vi "Data_get.vi"() -> ()   [LabVIEW 2009]
uses:
  <vilib>/Analysis/2dsp.llb/Real FFT.vi
  <vilib>/Analysis/NI_AALPro.lvlib
panel:
  in  "#steps":u32=1 min=1
  in  "f step (MHz)":dbl=0.0003 min=0.00025 max=67.0 step=1e-06 format="%#.12f"
  in  "ps/point":T1(ring)
  in  "ns/div":T2(ring)
  out "Current sweep":u32=1 min=1 max=1000 step=1
  in  "Ext":string="ccd"
  out "f cur. (MHz)":string
  in  "Name":string="trace"
  in  "Folder":path
  in  "#Sweeps":u32=1 min=1 max=1000 step=1
  in  "Ampl. (dBm)":dbl min=-135.0 max=30.0 step=0.5 format="%#_8g"
  in  "f start (MHz)":dbl=0.0003 min=0.00025 max=67.0 step=1e-06 format="%#.12f"
  in  "Start":bool
  in  "Quit":bool
  in  "E8257D VISA Port":refnum<visa-resource-name>="GPIB0::1::INSTR"
  out "read time (ms)":u32
  out "#points":u32
  out "Busy":bool
  in  "Repetition rate (Hz)":ext=2.5
  in  "Chirp start (MHz)":ext=2.5
  in  "Filter up to (MHz)":ext=2.5
  in  "Amount of averagings":u32=10
  out "Data":dbl[](array[numeric])
  out "XY Graph 5":cluster{ext[], dbl[]}(graph)
  out "FFT (Im)":dbl[](array[numeric])
  out "FFT (Re)":dbl[](array[numeric])
  out "Final array":ext[][](array[numeric])
  out "size(s)":i32
  out "Oscilloscope Data":dbl[](array[numeric])
  in  "Channel Number":u16=1
  out "Oscilloscope graph":dbl[](graph)
  in  "Stop":bool
  in  "TDS VISA Port":refnum<visa-resource-name>="GPIB0::1::INSTR"
  # "TDS6000"
  # "E8257D"
  # "File Storage"
  # "Control"
  # "Spectrum data"
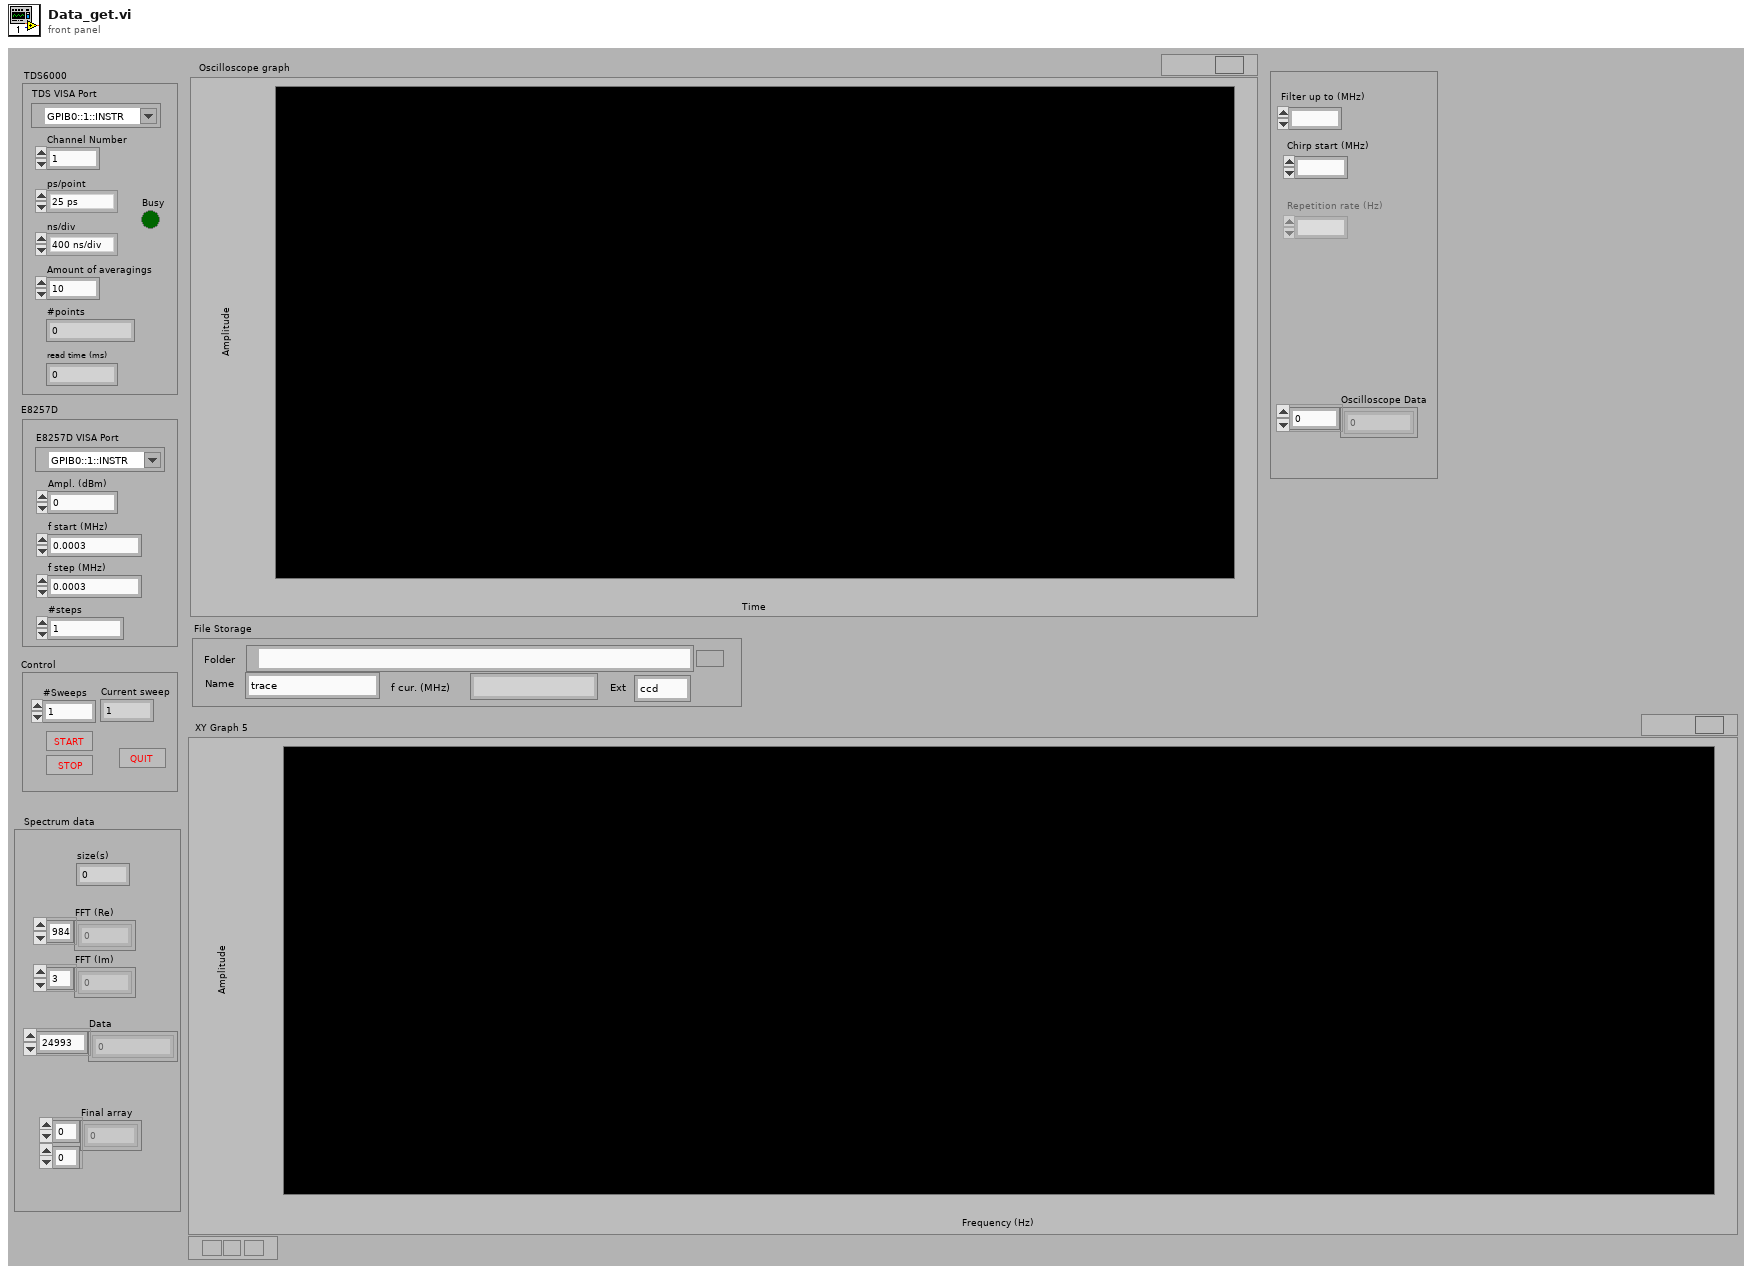
[diagram p1: front panel]
types:
  T1 = enum16{"25 ps", "50 ps", "100 ps", "200 ps", "400 ps", "800 ps", "2 ns"}
  T2 = enum16{"400 ns/div", "1 us/div", "2 us/div", "4 us/div", "10 us/div", "20 us/div"}
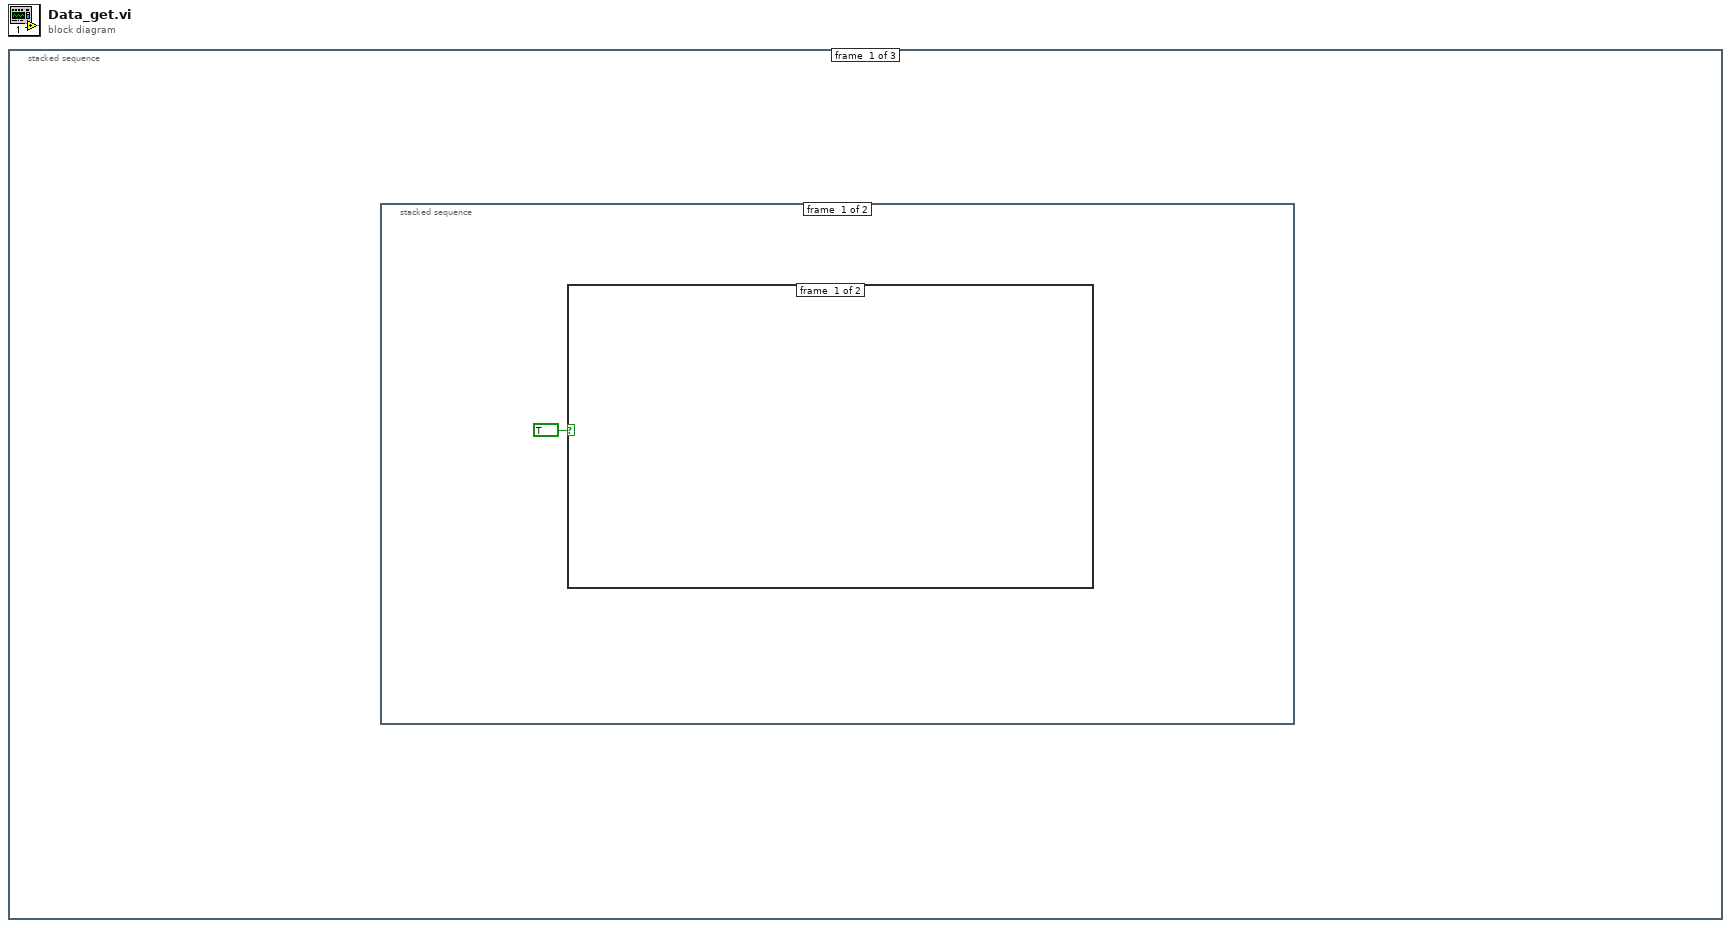
[diagram p0: block diagram]
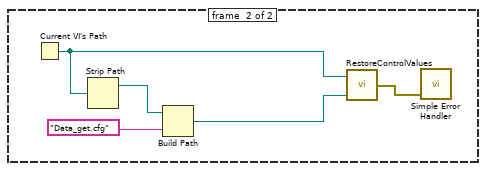
[diagram p2: hidden frame]
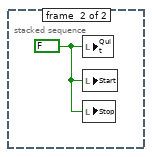
[diagram p3: hidden frame]
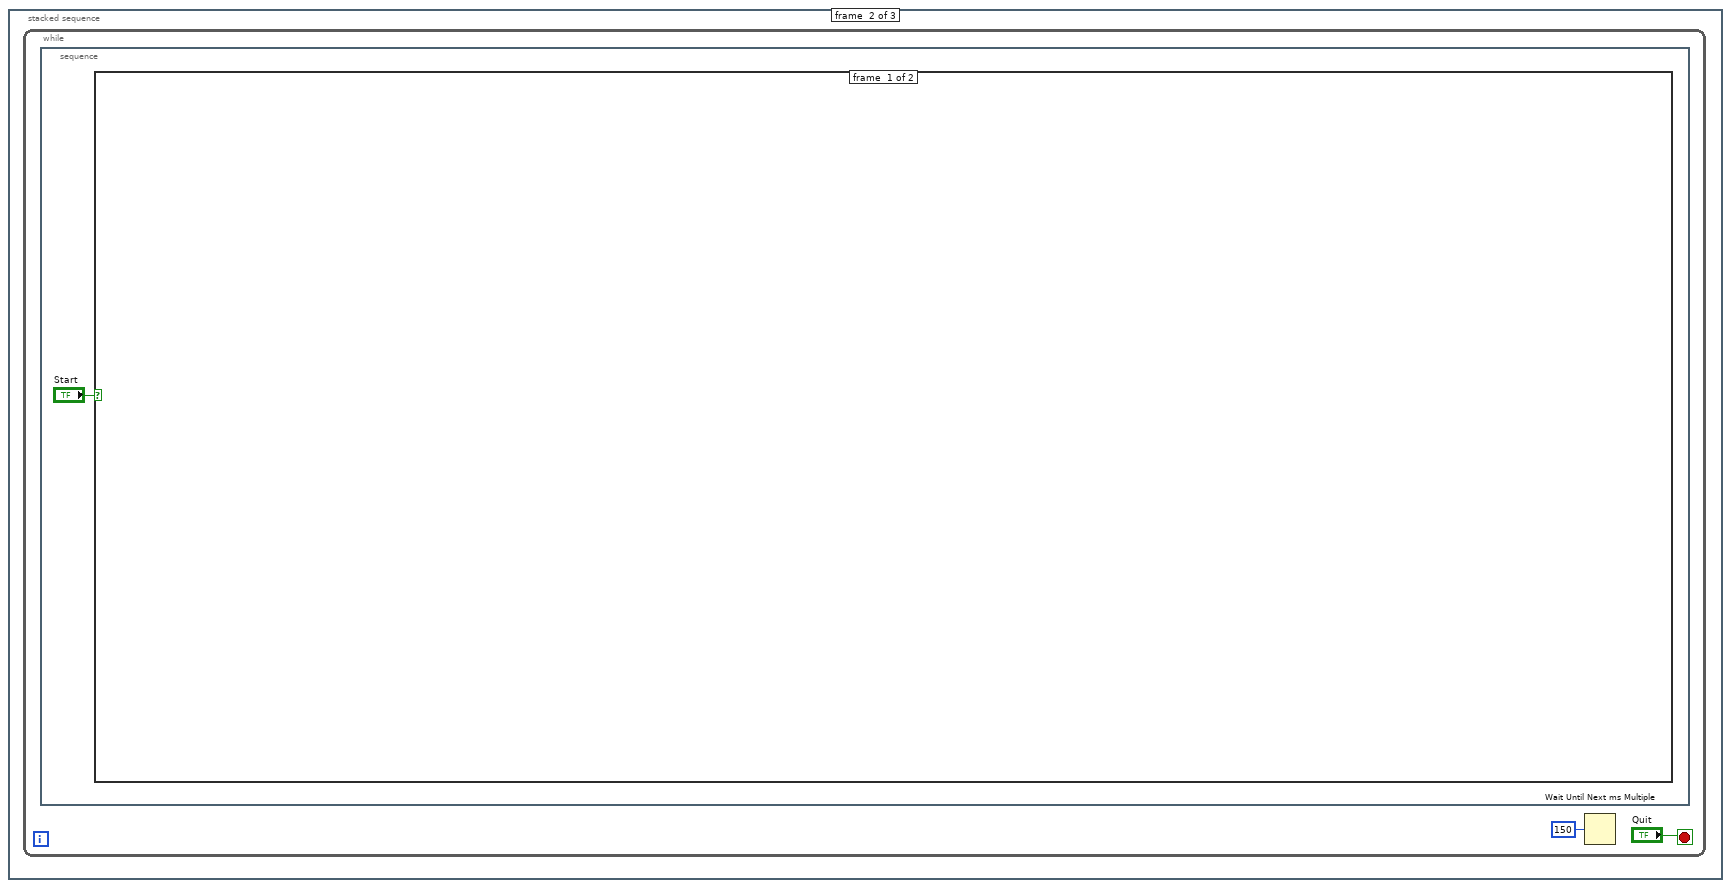
[diagram p4: hidden frame]
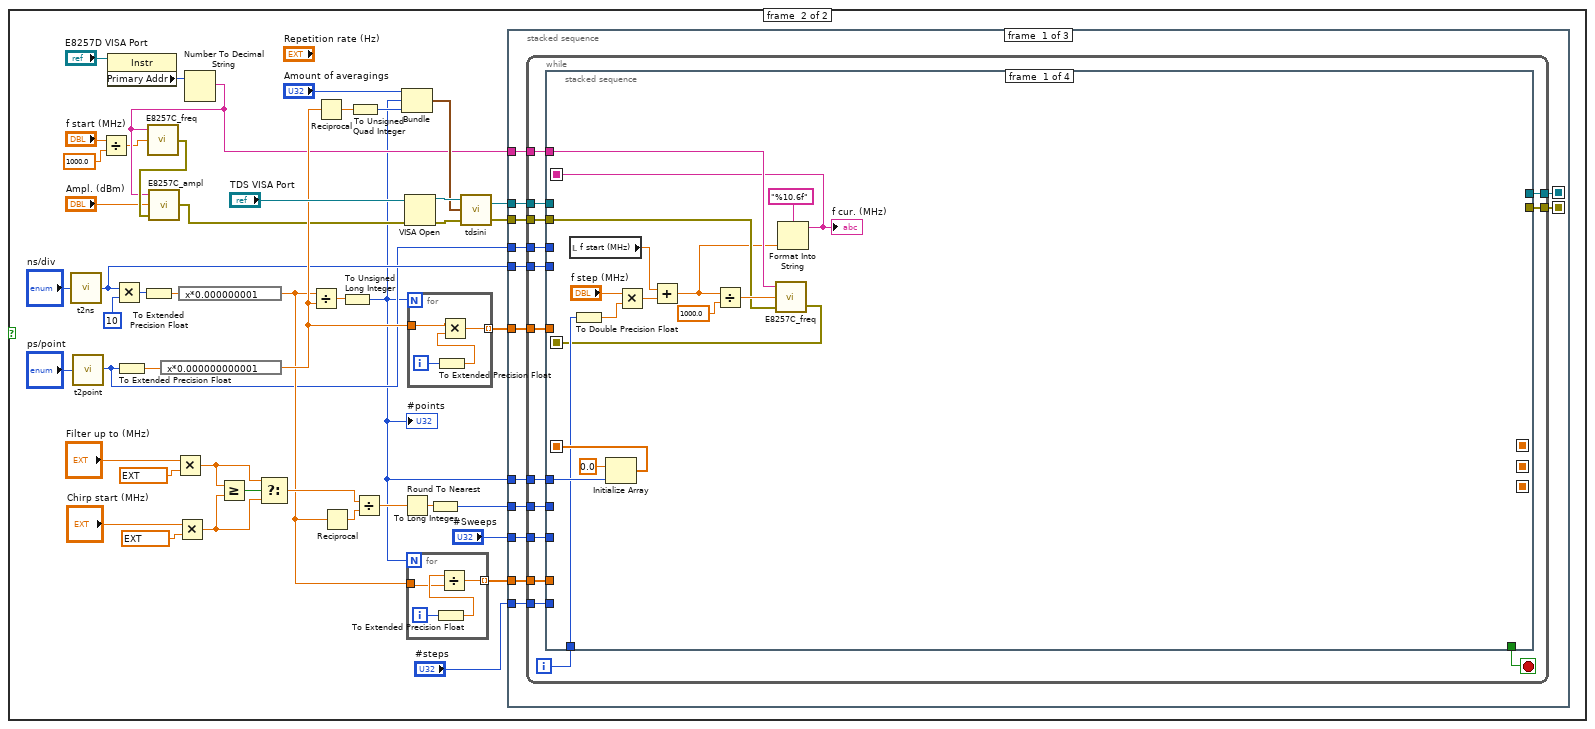
[diagram p5: hidden frame]
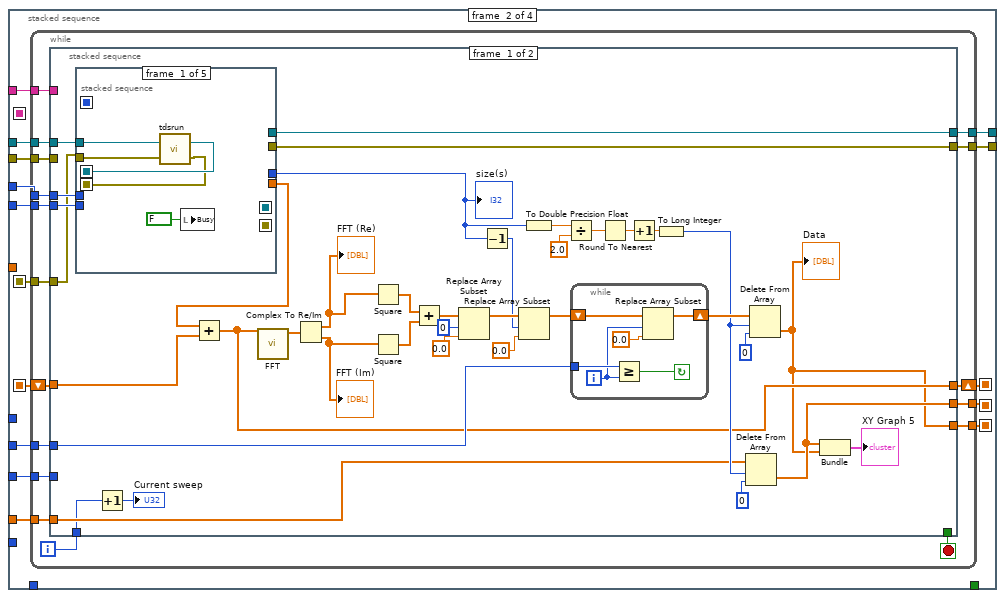
[diagram p6: hidden frame]
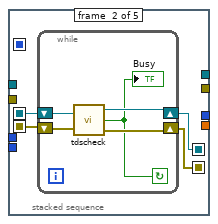
[diagram p7: hidden frame]
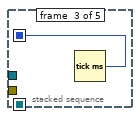
[diagram p8: hidden frame]
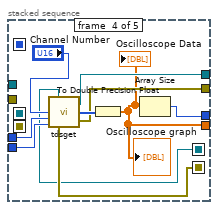
[diagram p9: hidden frame]
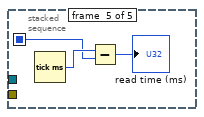
[diagram p10: hidden frame]
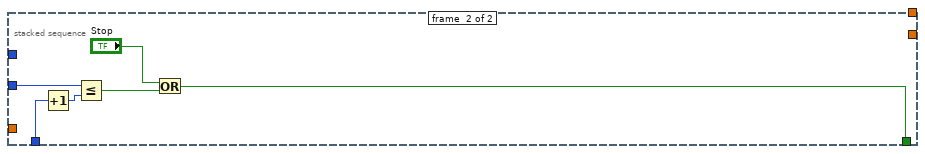
[diagram p11: hidden frame]
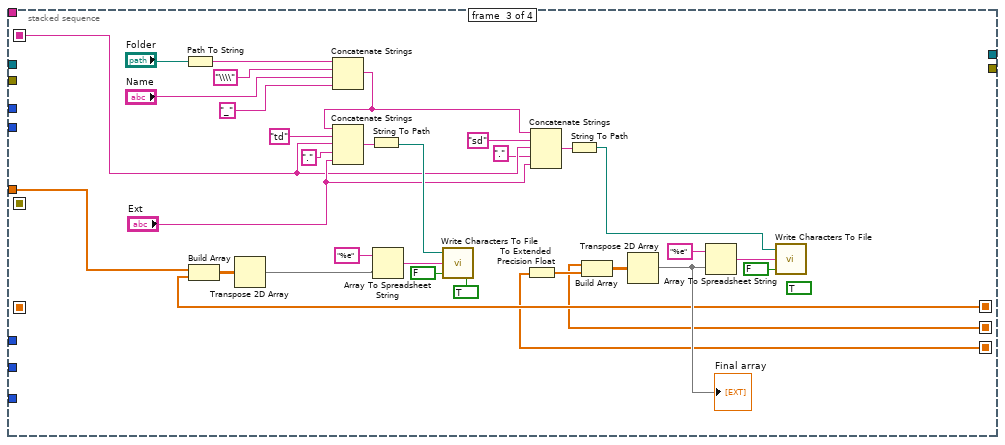
[diagram p12: hidden frame]
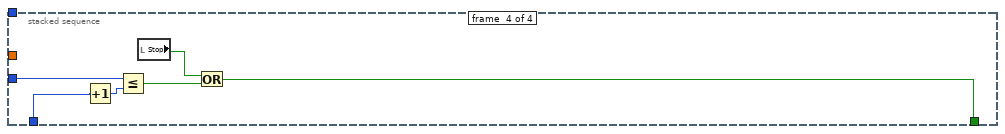
[diagram p13: hidden frame]
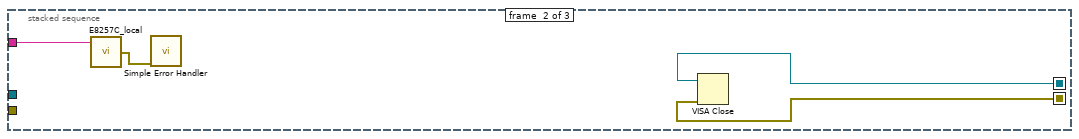
[diagram p14: hidden frame]
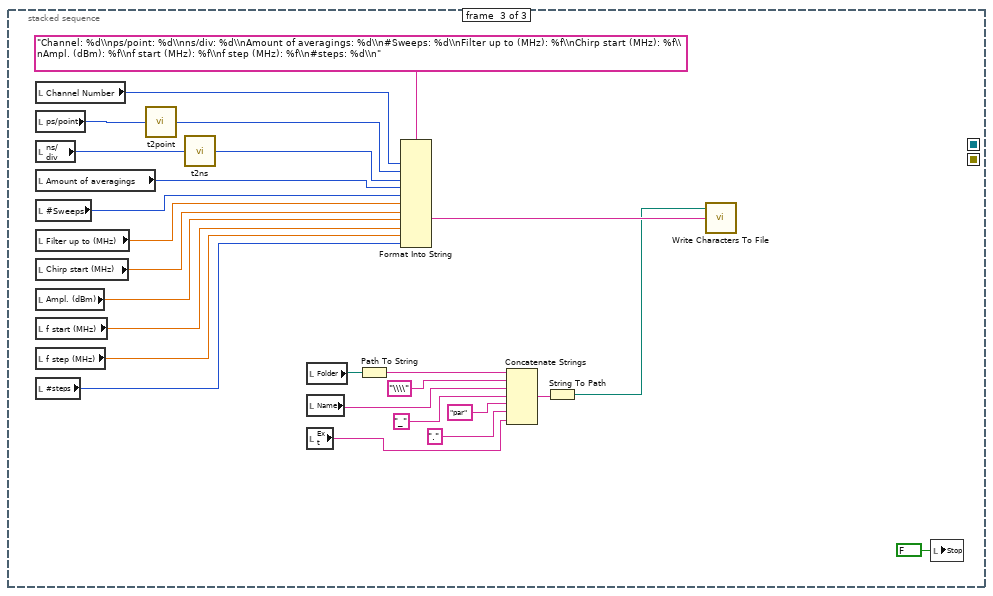
[diagram p15: hidden frame]
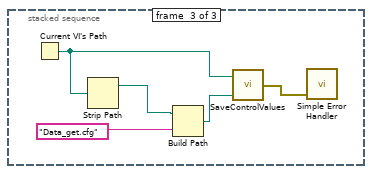
[diagram p16: hidden frame]
diagram:
  n1 = stacked-sequence {
    frame #0 {
      n2 = stacked-sequence {
        frame #0 {
          n3 = case shown="True" TRUE {
            frame #0 {
            }
            frame #1 {
              n4 = Current VI's Path() -> (path=w2:path)
              n5 = Strip Path(path=w2) -> (stripped path=w3:path)  [unwired: 1 out]
              n6 = Build Path(base path=w3, name or relative path="Data_get.cfg") -> (appended path=w5:path)
              n7 = call "RestoreControlValues.vi"("file path"=w5, "vi path"=w2) -> ("error out"=w4:errorcluster)
              n8 = call <vilib>:"Simple Error Handler.vi"("error in (no error)"=w4) -> ()  [unwired: 4 in, 5 out]
            }
          }
        }
        frame #1 {
          w7 = FALSE ("Quit")
          n9 = local write "Quit"(w7) -> ()
          n10 = local write "Start"(w7) -> ()
          n11 = local write "Stop"(w7) -> ()
        }
      }
    }
    frame #1 {
      n12 = while {
        stop <- "Quit" stop-if-true
        n13 = stacked-sequence {
          frame #0 {
            n14 = case shown="True" "Start" {
              frame #0 {
              }
              frame #1 {
                n15 = call "t2ns.vi"("t/div"="ns/div") -> ("ns/div"=w16:u32)
                n16 = call "t2point.vi"("t/point"="ps/point") -> ("ps/point"=w14:u32)
                n17 = Divide(x="f start (MHz)", y=1000.0) -> (x/y=w19:dbl)
                n18 = property class="Instr"(reference="E8257D VISA Port") -> ("Primary Addr"=w26:u16)  [unwired: 1 in, 2 out]
                n19 = Multiply(x=w16, y=u32 10) -> (x*y=w50:u32)
                n20 = To Extended Precision Float(1:w14) -> (0:w47:ext)
                n21 = To Extended Precision Float(1:w50) -> (0:w48:ext)
                n22 = expression code="x*0.000000000001"(w47) -> (w32:ext)
                n23 = Multiply(x="Filter up to (MHz)", y=ext 1000000.0) -> (x*y=w38:ext)
                n24 = Multiply(x="Chirp start (MHz)", y=ext 1000000.0) -> (x*y=w35:ext)
                n25 = expression code="x*0.000000001"(w48) -> (w28:ext)
                n26 = Number To Decimal String(number=w26) -> (decimal integer string=w23:string)  [unwired: 1 in]
                n27 = call "E8257C_freq.vi"("Frequency GHz"=w19, "GPIB address"=w23) -> ("error out"=w24:errorcluster)  [unwired: 1 in]
                n28 = call "E8257C_ampl.vi"("error in"=w24, "Amplitude dBm"="Ampl. (dBm)", "GPIB address"=w23) -> ("error out"=w22:errorcluster)
                n29 = Greater Or Equal?(x=w38, y=w35) -> (x >= y?=w46:bool)
                n30 = Select(t=w38, s=w46, f=w35) -> (s? t:f=w44:ext)
                n31 = Divide(x=w28, y=w32) -> (x/y=w49:ext)
                n32 = Reciprocal(x=w32) -> (1/x=w30:ext)
                n33 = Reciprocal(x=w28) -> (1/x=w45:ext)
                n34 = To Unsigned Long Integer(number=w49) -> (unsigned 32bit integer=w12:u32)
                "#points" <- w12
                n35 = To Unsigned Quad Integer(1:w30) -> (0:w31:u64)
                n36 = Divide(x=w44, y=w45) -> (x/y=w43:ext)
                n37 = Bundle("Amount of averagings"="Amount of averagings", w12, w31) -> (w33:cluster{"Amount of averagings ":u32, u32, u64})  [unwired: 1 in]
                n38 = Round To Nearest(number=w43) -> (nearest integer value=w42:ext)
                n39 = VISA Open(error in (no error)=w22, VISA resource name="TDS VISA Port") -> (VISA resource name=w53:refnum<visa-resource-name>, error out=w54:errorcluster)  [unwired: 3 in]
                n40 = for {
                  N: w12 -> [_]
                  tunnel: w28 -> [w279]
                  tunnel: [w281] -> w29 mode=indexing
                  i -> [w282]
                  n41 = To Extended Precision Float(1:w282) -> (0:w280:ext)
                  n42 = Divide(x=w280, y=w279) -> (x/y=w281:ext)
                }
                n43 = for {
                  N: w12 -> [_]
                  tunnel: w32 -> [w284]
                  tunnel: [w283] -> w17 mode=indexing
                  i -> [w286]
                  n44 = To Extended Precision Float(1:w286) -> (0:w285:ext)
                  n45 = Multiply(x=w284, y=w285) -> (x*y=w283:ext)
                }
                n46 = To Long Integer(number=w42) -> (32bit integer=w41:i32)
                n47 = call "tdsini.vi"("Error In (No Error)"=w54, "Acq_par"=w33, "VISA Port In"=w53) -> ("Error Out"=w55:errorcluster, "VISA Port Out"=w56:refnum<visa-resource-name>)
                n48 = stacked-sequence {
                  seq-local: [w61 _ _] -> [_ w252 _]
                  seq-local: [w60 _ _] -> [_ w251 _]
                  tunnel: w56 -> [w69 _ _]
                  tunnel: w55 -> [w68 _ _]
                  tunnel: w14 -> [w67 _ _]
                  tunnel: w16 -> [w66 _ _]
                  tunnel: w41 -> [w65 _ _]
                  tunnel: w29 -> [w64 _ _]
                  tunnel: w23 -> [w63 w249 _]
                  tunnel: "#Sweeps" -> [w62 _ _]
                  tunnel: w17 -> [w57 _ _]
                  tunnel: w12 -> [w59 _ _]
                  tunnel: "#steps" -> [w58 _ _]
                  frame #0 {
                    n49 = while {
                      tunnel: w69 -> [w84]
                      tunnel: w68 -> [w83]
                      tunnel: w67 -> [w82]
                      tunnel: w66 -> [w81]
                      tunnel: w65 -> [w80]
                      tunnel: w64 -> [w79]
                      tunnel: w63 -> [w78]
                      tunnel: w62 -> [w77]
                      tunnel: [w76] -> w61
                      tunnel: [w75] -> w60
                      tunnel: w59 -> [w74]
                      tunnel: w58 -> [w72]
                      tunnel: w57 -> [w70]
                      i -> [w73]
                      stop <- w71 stop-if-true
                      n50 = stacked-sequence {
                        seq-local: [w99 _ _ _] -> [_ w105 _ _]
                        seq-local: [w88 _ _ _] -> [_ w104 _ _]
                        seq-local: [_ w103 _ _] -> [_ _ w217 _]
                        seq-local: [_ w102 _ _] -> [_ _ w216 _]
                        seq-local: [_ w101 _ _] -> [_ _ w215 _]
                        seq-local: [w85 _ _ _] -> [_ _ w212 _]
                        tunnel: w84 -> [_ w115 _ _]
                        tunnel: w83 -> [w89 w114 _ _]
                        tunnel: w82 -> [_ w113 _ _]
                        tunnel: w81 -> [_ w112 _ _]
                        tunnel: w80 -> [_ w111 _ _]
                        tunnel: w79 -> [_ w110 _ _]
                        tunnel: w78 -> [w90 w109 _ _]
                        tunnel: w77 -> [_ w108 _ _]
                        tunnel: [_ w107 _ _] -> w76
                        tunnel: [_ w106 _ _] -> w75
                        tunnel: w74 -> [w98 _ _ _]
                        tunnel: w73 -> [w93 _ _ w245]
                        tunnel: w72 -> [_ _ _ w244]
                        tunnel: [_ _ _ w243] -> w71
                        tunnel: w70 -> [_ _ w218 _]
                        frame #0 {
                          n51 = local read "f start (MHz)"() -> (w91:dbl)
                          n52 = To Double Precision Float(number=w93) -> (double precision float=w94:dbl)
                          n53 = Initialize Array(0.0 ("element"), w98) -> (w99:dbl[])
                          n54 = Multiply(x="f step (MHz)", y=w94) -> (x*y=w92:dbl)
                          n55 = Add(x=w91, y=w92) -> (x+y=w87:dbl)
                          n56 = Divide(x=w87, y=1000.0) -> (x/y=w97:dbl)
                          n57 = call "E8257C_freq.vi"("error in"=w89, "Frequency GHz"=w97, "GPIB address"=w90) -> ("error out"=w88:errorcluster)
                          n58 = Format Into String(format string="%10.6f", w87) -> (resulting string=w85:string)  [unwired: 2 in, 1 out]
                          "f cur. (MHz)" <- w85
                        }
                        frame #1 {
                          n59 = while {
                            tunnel: [w129] -> w106
                            tunnel: [w130] -> w107
                            tunnel: w114 -> [w131]
                            tunnel: w115 -> [w132]
                            tunnel: w113 -> [w128]
                            tunnel: w112 -> [w127]
                            tunnel: w110 -> [w125]
                            tunnel: w111 -> [w126]
                            tunnel: w109 -> [w122]
                            tunnel: w108 -> [w121]
                            shift-right: [w119] -> w103
                            shift-left: w105 -> [w120]
                            tunnel: [w118] -> w102
                            tunnel: [w117] -> w101
                            tunnel: w104 -> [w116]
                            i -> [w124]
                            stop <- w123 stop-if-true
                            n60 = stacked-sequence {
                              tunnel: w132 -> [w170 _]
                              tunnel: w131 -> [_ _]
                              tunnel: [w169 _] -> w130
                              tunnel: [w168 _] -> w129
                              tunnel: w128 -> [w167 _]
                              tunnel: w127 -> [w166 _]
                              tunnel: w126 -> [w152 _]
                              tunnel: w125 -> [w141 _]
                              tunnel: w124 -> [w134 w210]
                              tunnel: [_ w207] -> w123
                              tunnel: w122 -> [_ _]
                              tunnel: w121 -> [_ w206]
                              tunnel: w120 -> [w140 _]
                              tunnel: [w138 _] -> w119
                              tunnel: [w137 _] -> w118
                              tunnel: [w136 _] -> w117
                              tunnel: w116 -> [w133 _]
                              frame #0 {
                                n61 = stacked-sequence {
                                seq-local: [w179 _ _ _ _] -> [_ w185 _ _ _]
                                seq-local: [w178 _ _ _ _] -> [_ w184 _ _ _]
                                seq-local: [_ w182 _ _ _] -> [_ _ _ w193 _]
                                seq-local: [_ w183 _ _ _] -> [_ _ _ w192 _]
                                seq-local: [_ _ w191 _ _] -> [_ _ _ _ w203]
                                tunnel: w170 -> [w180 _ _ _ _]
                                tunnel: w133 -> [w181 _ _ _ _]
                                tunnel: [_ _ _ w200 _] -> w169
                                tunnel: [_ _ _ w199 _] -> w168
                                tunnel: w167 -> [_ _ _ w197 _]
                                tunnel: w166 -> [_ _ _ w196 _]
                                tunnel: [_ _ _ w195 _] -> w150
                                tunnel: [_ _ _ w194 _] -> w139
                                frame #0 {
                                n62 = call "tdsrun.vi"("Error In (No Error)"=w181, "VISA Port In"=w180) -> ("Error Out"=w178:errorcluster, "VISA Port Out"=w179:refnum<visa-resource-name>)
                                n63 = local write "Busy"(FALSE ("Busy")) -> ()
                                }
                                frame #1 {
                                n64 = while {
                                shift-right: [w188] -> w183
                                shift-left: w185 -> [w189]
                                shift-right: [w187] -> w182
                                shift-left: w184 -> [w190]
                                stop <- w186 continue-if-true
                                n65 = call "tdscheck.vi"("VISA Port In"=w189, "Error In (No Error)"=w190) -> ("VISA Port Out"=w188:refnum<visa-resource-name>, "busy"=w186:bool, "Error Out"=w187:errorcluster)
                                "Busy" <- w186
                                }
                                }
                                frame #2 {
                                n66 = Tick Count (ms)() -> (millisecond timer value=w191:u32)
                                }
                                frame #3 {
                                n67 = call "tdsget.vi"("VISA Port In"=w192, "Channel Number"="Channel Number", "ps/point"=w197, "ns/div"=w196, "Error In (No Error)"=w193) -> ("VISA Port Out"=w200:refnum<visa-resource-name>, "TDS Data"=w201:u16[], "Error Out"=w199:errorcluster)  [unwired: 8 in]
                                n68 = To Double Precision Float(number=w201) -> (double precision float=w194:dbl[])
                                "Oscilloscope graph" <- w194
                                "Oscilloscope Data" <- w194
                                n69 = Array Size(array=w194) -> (size(s)=w195:i32)
                                }
                                frame #4 {
                                n70 = Tick Count (ms)() -> (millisecond timer value=w204:u32)
                                n71 = Subtract(x=w204, y=w203) -> (x-y=→"read time (ms)":u32)
                                }
                                }
                                "size(s)" <- w150
                                n72 = Increment(x=w134) -> (x+1=→"Current sweep":i32)
                                n73 = Add(x=w139, y=w140) -> (x+y=w138:dbl[])
                                n74 = call-poly <vilib>:"FFT.vi"("X"=w138) -> ("FFT {X}"=w165:cdb[])  [unwired: 9 in, 1 out]
                                n75 = Complex To Re/Im(x + iy=w165) -> (x=w164:dbl[], y=w163:dbl[])
                                "FFT (Re)" <- w164
                                "FFT (Im)" <- w163
                                n76 = Square(x=w164) -> (x^2=w162:dbl[])
                                n77 = Square(x=w163) -> (x^2=w161:dbl[])
                                n78 = Add(x=w162, y=w161) -> (x+y=w157:dbl[])
                                n79 = Replace Array Subset(array=w157, new element=0.0 ("new element/subarray"), index=0) -> (w156:dbl[])
                                n80 = Decrement(x=w150) -> (x-1=w155:i32)
                                n81 = Replace Array Subset(array=w156, new element=0.0 ("new element/subarray"), index=w155) -> (w153:dbl[])
                                n82 = To Double Precision Float(number=w150) -> (double precision float=w149:dbl)
                                n83 = Divide(x=w149, y=2.0) -> (x/y=w147:dbl)
                                n84 = while {
                                tunnel: w152 -> [w175]
                                shift-right: [w173] -> w151
                                shift-left: w153 -> [w174]
                                i -> [w172]
                                stop <- w176 continue-if-true
                                n85 = Greater Or Equal?(x=w175, y=w172) -> (x >= y?=w176:bool)
                                n86 = Replace Array Subset(array=w174, new element=0.0 ("new element/subarray"), index=w172) -> (w173:dbl[])
                                }
                                n87 = Round To Nearest(number=w147) -> (nearest integer value=w146:dbl)
                                n88 = Increment(x=w146) -> (x+1=w145:dbl)
                                n89 = To Long Integer(number=w145) -> (32bit integer=w142:i32)
                                n90 = Delete From Array(array=w141, length=w142, index=0) -> (deleted portion=w137:ext[])  [unwired: 1 out]
                                n91 = Delete From Array(array=w151, length=w142, index=0) -> (deleted portion=w136:dbl[])  [unwired: 1 out]
                                "Data" <- w136
                                n92 = Bundle(w137, w136) -> (→"XY Graph 5":cluster{ext[], dbl[]})  [unwired: 1 in]
                              }
                              frame #1 {
                                n93 = Increment(x=w210) -> (x+1=w205:i32)
                                n94 = Less Or Equal?(x=w206, y=w205) -> (x <= y?=w209:bool)
                                n95 = Or(x="Stop", y=w209) -> (x .or. y?=w207:bool)
                              }
                            }
                          }
                        }
                        frame #2 {
                          (unwired) TRUE
                          n96 = Path To String(path="Folder") -> (string=w236:string)
                          n97 = Build Array(w218, w217) -> (w237:ext[][])
                          n98 = Transpose 2D Array(2D array=w237) -> (transposed array=w224:ext[][])
                          n99 = Concatenate Strings(w236, "\\\\" ("string"), "Name", "_") -> (w220:string)
                          n100 = Concatenate Strings(w220, "td", w212, ".", "Ext") -> (w230:string)
                          n101 = String To Path(string=w230) -> (path=w225:path)
                          n102 = Array To Spreadsheet String(array=w224, 3:"%e") -> (spreadsheet string=w227:string)  [unwired: 1 in]
                          n103 = call <vilib>:"Write Characters To File.vi"("convert eol? (no:F)"=TRUE, "append to file? (new file:F)"=FALSE, "character string"=w227, "file path (dialog if empty)"=w225) -> ()  [unwired: 1 in, 1 out]
                          n104 = To Extended Precision Float(1:w215) -> (0:w238:ext[])
                          n105 = Concatenate Strings(w220, "sd", w212, ".", "Ext") -> (w222:string)
                          n106 = String To Path(string=w222) -> (path=w221:path)
                          n107 = Build Array(w216, w238) -> (w214:ext[][])
                          n108 = Transpose 2D Array(2D array=w214) -> (transposed array=w241:ext[][])
                          "Final array" <- w241
                          n109 = Array To Spreadsheet String(array=w241, 3:"%e") -> (spreadsheet string=w239:string)  [unwired: 1 in]
                          n110 = call <vilib>:"Write Characters To File.vi"("append to file? (new file:F)"=FALSE, "character string"=w239, "file path (dialog if empty)"=w221) -> ()  [unwired: 2 in, 1 out]
                        }
                        frame #3 {
                          n111 = Increment(x=w245) -> (x+1=w247:i32)
                          n112 = Less Or Equal?(x=w244, y=w247) -> (x <= y?=w248:bool)
                          n113 = local read "Stop"() -> (w246:bool)
                          n114 = Or(x=w246, y=w248) -> (x .or. y?=w243:bool)
                        }
                      }
                    }
                  }
                  frame #1 {
                    n115 = call "E8257C_local.vi"("GPIB address"=w249) -> ("error out"=w250:errorcluster)  [unwired: 1 in]
                    n116 = call <vilib>:"Simple Error Handler.vi"("error in (no error)"=w250) -> ()  [unwired: 4 in, 5 out]
                    n117 = VISA Close(VISA resource name=w252, error in (no error)=w251) -> ()  [unwired: 1 out]
                  }
                  frame #2 {
                    n118 = local read "Channel Number"() -> (w276:u16)
                    n119 = local read "ps/point"() -> (w275:T1)
                    n120 = local read "ns/div"() -> (w274:T2)
                    n121 = local read "Amount of averagings"() -> (w273:u32)
                    n122 = local read "#Sweeps"() -> (w271:u32)
                    n123 = local read "Filter up to (MHz)"() -> (w270:ext)
                    n124 = local read "Chirp start (MHz)"() -> (w269:ext)
                    n125 = local read "Ampl. (dBm)"() -> (w268:dbl)
                    n126 = local read "f start (MHz)"() -> (w265:dbl)
                    n127 = local read "f step (MHz)"() -> (w264:dbl)
                    n128 = local read "#steps"() -> (w263:u32)
                    n129 = call "t2point.vi"("t/point"=w275) -> ("ps/point"=w266:u32)
                    n130 = call "t2ns.vi"("t/div"=w274) -> ("ns/div"=w267:u32)
                    n131 = local read "Folder"() -> (w259:path)
                    n132 = local read "Name"() -> (w258:string)
                    n133 = local read "Ext"() -> (w255:string)
                    n134 = Path To String(path=w259) -> (string=w262:string)
                    n135 = Format Into String(format string="Channel: %d\\nps/point: %d\\nns/div: %d\\nAmount of averagings: %d\\n#Sweeps: %d\\nFilter up to (MHz): %f\\nChirp start (MHz): %f\\nAmpl. (dBm): %f\\nf start (MHz): %f\\nf step (MHz): %f\\n#steps: %d\\n", w276, w266, w267, w273, w271, w270, w269, w268, w265, w264, w263) -> (resulting string=w278:string)  [unwired: 2 in, 1 out]
                    n136 = Concatenate Strings(w262, "\\\\" ("string"), w258, "_", "par", ".", w255) -> (w254:string)
                    n137 = String To Path(string=w254) -> (path=w253:path)
                    n138 = call <vilib>:"Write Characters To File.vi"("character string"=w278, "file path (dialog if empty)"=w253) -> ()  [unwired: 3 in, 1 out]
                    n139 = local write "Stop"(FALSE ("Stop")) -> ()
                  }
                }
              }
            }
          }
        }
        n140 = Wait Until Next ms Multiple(millisecond multiple=u32 150) -> ()  [unwired: 1 out]
      }
    }
    frame #2 {
      n141 = Current VI's Path() -> (path=w287:path)
      n142 = Strip Path(path=w287) -> (stripped path=w288:path)  [unwired: 1 out]
      n143 = Build Path(base path=w288, name or relative path="Data_get.cfg") -> (appended path=w290:path)
      n144 = call "SaveControlValues.vi"("file path"=w290, "vi path"=w287) -> ("error out"=w289:errorcluster)
      n145 = call <vilib>:"Simple Error Handler.vi"("error in (no error)"=w289) -> ()  [unwired: 4 in, 5 out]
    }
  }
